vi "Check New Clipboard Value.vi"(8 "error in (no error)":errorcluster) -> (1 "New Value?":bool, 2 "Values":dbl[][](array[numeric]), 3 "Read From Clipboard":string)   [LabVIEW 2019]
panel:
  out "error out":errorcluster
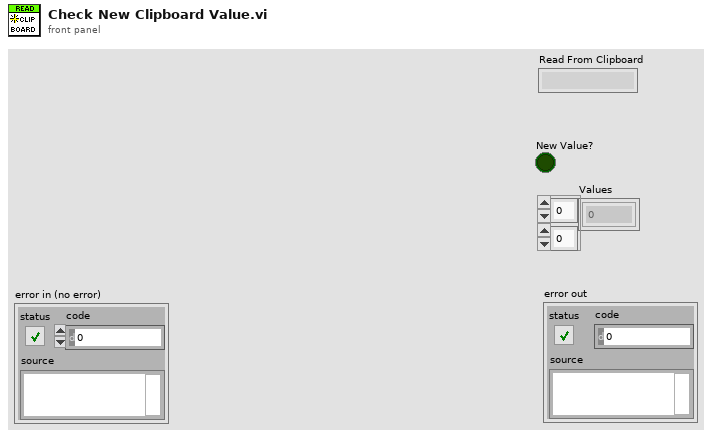
[diagram p1: front panel]
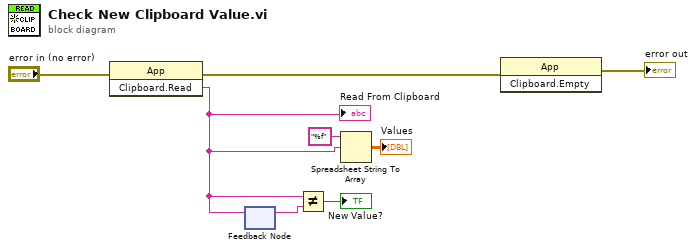
[diagram p0: block diagram]
diagram:
  n1 = invoke class="App" method="Clipboard.Read"(error in="error in (no error)") -> (error out=w1:errorcluster, "Read Clipbrd"=w7:string)  [unwired: 2 in, 1 out]
  "Read From Clipboard" <- w7
  n2 = feedback #1() -> (w4:string)  [unwired: 1 in]
  n3 = feedback-in #1(w7) -> ()
  n4 = Not Equal?(x=w7, y=w4) -> (x != y?=→"New Value?":bool)
  n5 = Spreadsheet String To Array(format string="%f", spreadsheet string=w7) -> (array=→"Values":dbl[][])  [unwired: 2 in]
  n6 = invoke class="App" method="Clipboard.Empty"(error in=w1) -> (error out=→"error out":errorcluster)  [unwired: 2 in, 2 out]
